vi "Array_to_cluster_sequence_SubVI_v1.vi"(1 "Array":cluster{"Timing 0":dbl[]}[](array[cluster])) -> (0 "Sequence":T1)   [LabVIEW 2021]
uses:
  Addons/DAQ_Pulse_Gen/DAQ_Control_1.ctl
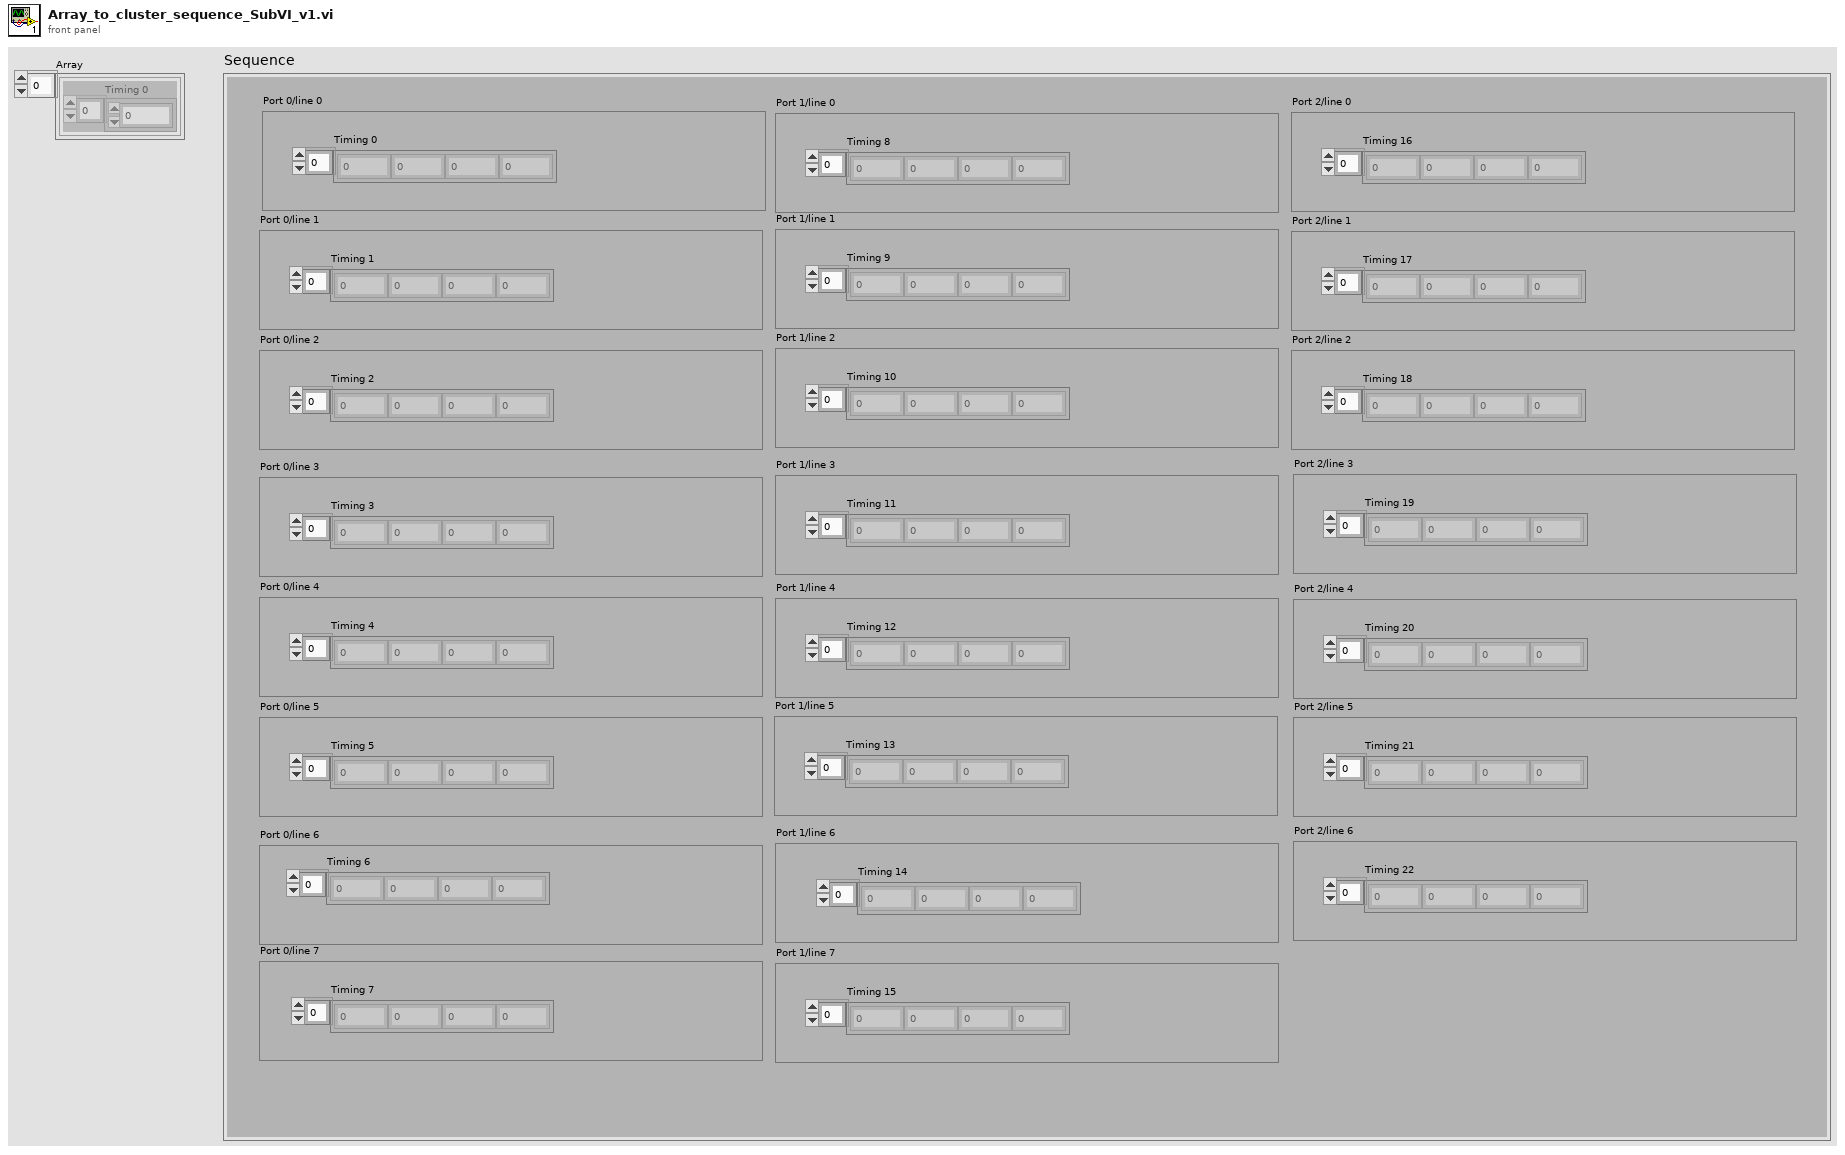
[diagram p1: front panel]
types:
  T1 = typedef "DAQ_Control_1.ctl" = cluster{"Port 2/line 6":cluster{"Timing 22":dbl[]}, "Port 2/line 5":cluster{"Timing 21":dbl[]}, "Port 2/line 4":cluster{"Timing 20":dbl[]}, "Port 2/line 3":cluster{"Timing 19":dbl[]}, "Port 2/line 2":cluster{"Timing 18":dbl[]}, "Port 2/line 1":cluster{"Timing 17":dbl[]}, "Port 2/line 0":cluster{"Timing 16":dbl[]}, "Port 1/line 7":cluster{"Timing 15":dbl[]}, "Port 1/line 6":cluster{"Timing 14":dbl[]}, "Port 1/line 5":cluster{"Timing 13":dbl[]}, "Port 1/line 4":cluster{"Timing 12":dbl[]}, "Port 1/line 3":cluster{"Timing 11":dbl[]}, "Port 1/line 2":cluster{"Timing 10":dbl[]}, "Port 1/line 1":cluster{"Timing 9":dbl[]}, "Port 1/line 0":cluster{"Timing 8":dbl[]}, "Port 0/line 7":cluster{"Timing 7\n":dbl[]}, "Port 0/line 6":cluster{"Timing 6\n":dbl[]}, "Port 0/line 5":cluster{"Timing 5\n":dbl[]}, "Port 0/line 4":cluster{"Timing 4\n":dbl[]}, "Port 0/line 3":cluster{"Timing 3\n":dbl[]}, "Port 0/line 2":cluster{"Timing 2":dbl[]}, "Port 0/line 1":cluster{"Timing 1\n":dbl[]}, "Port 0/line 0":cluster{"Timing 0":dbl[]}}
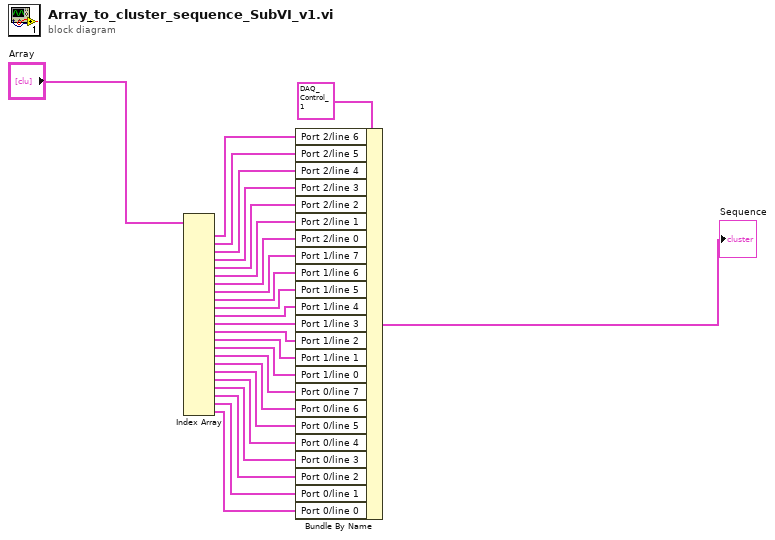
[diagram p0: block diagram]
diagram:
  n1 = Index Array(array="Array") -> (element #1=w3:cluster{"Timing 0":dbl[]}, element #2=w5:cluster{"Timing 0":dbl[]}, element #3=w4:cluster{"Timing 0":dbl[]}, element #4=w6:cluster{"Timing 0":dbl[]}, element #5=w7:cluster{"Timing 0":dbl[]}, element #6=w8:cluster{"Timing 0":dbl[]}, element #7=w9:cluster{"Timing 0":dbl[]}, element #8=w11:cluster{"Timing 0":dbl[]}, element #9=w12:cluster{"Timing 0":dbl[]}, element #10=w13:cluster{"Timing 0":dbl[]}, element #11=w14:cluster{"Timing 0":dbl[]}, element #12=w15:cluster{"Timing 0":dbl[]}, element #13=w16:cluster{"Timing 0":dbl[]}, element #14=w17:cluster{"Timing 0":dbl[]}, element #15=w18:cluster{"Timing 0":dbl[]}, element #16=w19:cluster{"Timing 0":dbl[]}, element #17=w20:cluster{"Timing 0":dbl[]}, element #18=w21:cluster{"Timing 0":dbl[]}, element #19=w22:cluster{"Timing 0":dbl[]}, element #20=w23:cluster{"Timing 0":dbl[]}, element #21=w24:cluster{"Timing 0":dbl[]}, element #22=w25:cluster{"Timing 0":dbl[]}, element #23=w26:cluster{"Timing 0":dbl[]})  [unwired: 23 in]
  n2 = Bundle By Name(cluster=T1 {"Port 2/line 6"={"Timing 22"=[]}, "Port 2/line 5"={"Timing 21"=[]}, "Port 2/line 4"={"Timing 20"=[]}, "Port 2/line 3"={"Timing 19"=[]}, "Port 2/line 2"={"Timing 18"=[]}, "Port 2/line 1"={"Timing 17"=[]}, "Port 2/line 0"={"Timing 16"=[]}, "Port 1/line 7"={"Timing 15"=[]}, "Port 1/line 6"={"Timing 14"=[]}, "Port 1/line 5"={"Timing 13"=[]}, "Port 1/line 4"={"Timing 12"=[]}, "Port 1/line 3"={"Timing 11"=[]}, "Port 1/line 2"={"Timing 10"=[]}, "Port 1/line 1"={"Timing 9"=[]}, "Port 1/line 0"={"Timing 8"=[]}, "Port 0/line 7"={"Timing 7\n"=[]}, "Port 0/line 6"={"Timing 6\n"=[]}, "Port 0/line 5"={"Timing 5\n"=[]}, "Port 0/line 4"={"Timing 4\n"=[]}, "Port 0/line 3"={"Timing 3\n"=[]}, "Port 0/line 2"={"Timing 2"=[]}, "Port 0/line 1"={"Timing 1\n"=[]}, "Port 0/line 0"={"Timing 0"=[]}} ("Sequence"), "Port 2/line 6"=w3, "Port 2/line 5"=w5, "Port 2/line 4"=w4, "Port 2/line 3"=w6, "Port 2/line 2"=w7, "Port 2/line 1"=w8, "Port 2/line 0"=w9, "Port 1/line 7"=w11, "Port 1/line 6"=w12, "Port 1/line 5"=w13, "Port 1/line 4"=w14, "Port 1/line 3"=w15, "Port 1/line 2"=w16, "Port 1/line 1"=w17, "Port 1/line 0"=w18, "Port 0/line 7"=w19, "Port 0/line 6"=w20, "Port 0/line 5"=w21, "Port 0/line 4"=w22, "Port 0/line 3"=w23, "Port 0/line 2"=w24, "Port 0/line 1"=w25, "Port 0/line 0"=w26) -> (→"Sequence":T1)
